vi "sub_互相关.vi"(5 "互相关点数":i32=5, 6 "y":dbl[](array[numeric])=[1.0, 2.0, 3.0, 4.0, 5.0, 6.0], 7 "x":dbl[](array[numeric])=[1.0, 2.0, 3.0, 4.0, 5.0, 6.0]) -> (1 "最大值":dbl, 2 "中心偏移":i32, 3 "输出数组":dbl[](array[numeric]))   [LabVIEW 2015]
panel:
  out "输出数组图形":dbl[](graph)
  out "最大索引":i32
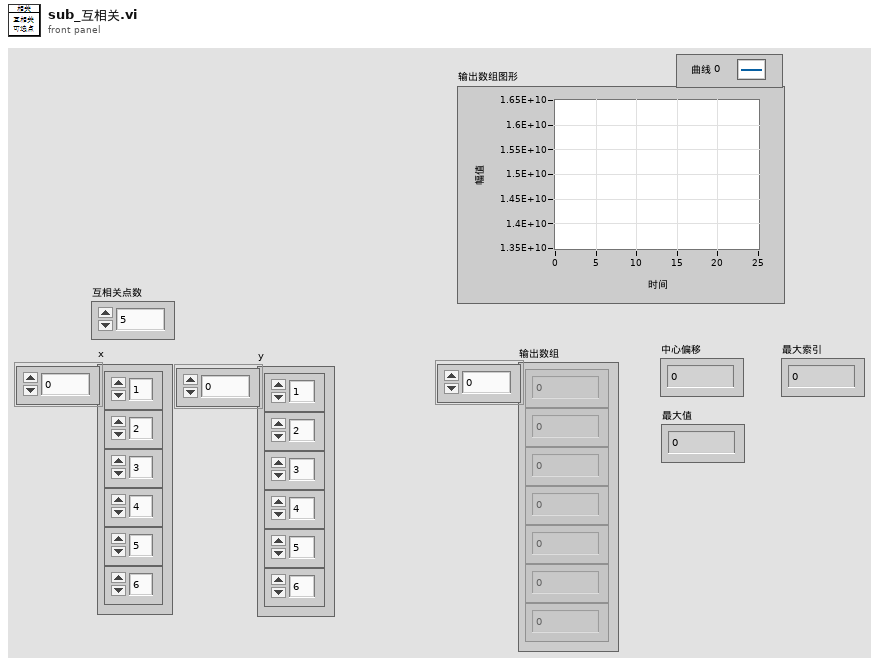
[diagram p1: front panel]
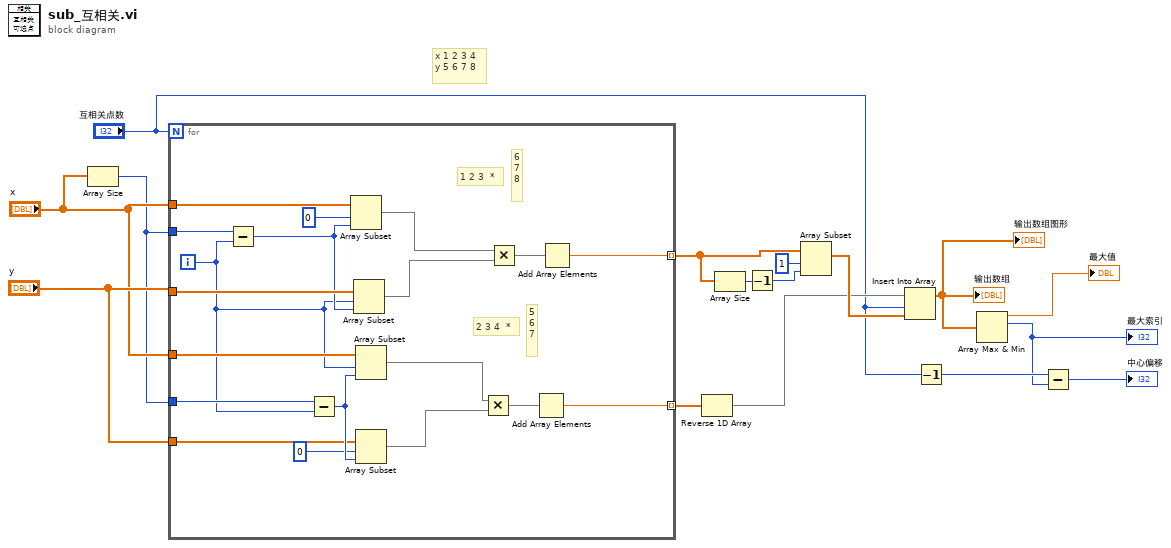
[diagram p0: block diagram]
diagram:
  # "x 1 2 3 4\ny 5 6 7 8"
  n1 = Array Size(array="x") -> (size(s)=w8:i32)
  n2 = for {
    N: "互相关点数" -> [_]
    tunnel: "x" -> [w35]
    tunnel: w8 -> [w34]
    tunnel: "y" -> [w33]
    tunnel: [w28] -> w13 mode=indexing
    tunnel: "x" -> [w26]
    tunnel: "y" -> [w25]
    tunnel: [w21] -> w15 mode=indexing
    tunnel: w8 -> [w20]
    i -> [w19]
    # "5\n6\n7"
    # "2 3 4  *"
    # "6\n7\n8"
    # "1 2 3  *"
    n3 = Subtract(x=w34, y=w19) -> (x-y=w32:i32)
    n4 = Subtract(x=w20, y=w19) -> (x-y=w27:i32)
    n5 = Array Subset(array=w35, index=0 ("索引"), length=w32) -> (w30:dbl[])
    n6 = Array Subset(array=w33, index=w19, length=w32) -> (w31:dbl[])
    n7 = Array Subset(array=w26, index=w19, length=w27) -> (w23:dbl[])
    n8 = Array Subset(array=w25, index=0 ("索引"), length=w27) -> (w22:dbl[])
    n9 = Multiply(x=w23, y=w22) -> (x*y=w24:dbl[])
    n10 = Multiply(x=w30, y=w31) -> (x*y=w29:dbl[])
    n11 = Add Array Elements(numeric array=w24) -> (sum=w21:dbl)
    n12 = Add Array Elements(numeric array=w29) -> (sum=w28:dbl)
  }
  n13 = Reverse 1D Array(array=w15) -> (reversed array=w4:dbl[])
  n14 = Array Size(array=w13) -> (size(s)=w12:i32)
  n15 = Decrement(x=w12) -> (x-1=w11:i32)
  n16 = Array Subset(array=w13, index=1 ("索引"), length=w11) -> (w10:dbl[])
  n17 = Insert Into Array(array=w4, index="互相关点数", new element=w10) -> (w5:dbl[])
  "输出数组" <- w5
  "输出数组图形" <- w5
  n18 = Decrement(x="互相关点数") -> (x-1=w2:i32)
  n19 = Array Max & Min(array=w5) -> (max value=→"最大值":dbl, max index (indices)=w1:i32)  [unwired: 2 out]
  "最大索引" <- w1
  n20 = Subtract(x=w2, y=w1) -> (x-y=→"中心偏移":i32)
